vi "Load SVG Image (Path).vi"(8 "error in (no error)":errorcluster, 10 "Scale (1)":dbl=1.0, 11 "Path In":path) -> (0 "error out":errorcluster, 2 "Image":T1, 3 "Path Out":path)   [LabVIEW 2020, in "G-Image.lvlib"]
doc: "Load a Scalable Vector Graphics (SVG) image file from disk, and return it as a LabVIEW picture. The SVG is loaded assuming using 96 DPI and px units. Use the <b>Scale</b> input to adjust the size of the image being loaded.\n\nThe input can be a standard path type, a UTF-8 encoded path string, or a byte array."
uses:
  G-Image.lvlib
  <vilib>/picture/picture.llb/imagedata.ctl
  Private/Debug Path.vi
  Private/Result To Error.vi
  <vilib>/Utility/file.llb/Application Directory.vi
  <vilib>/Utility/error.llb/Error Cluster From Error Code.vi
  Private/Copy Image To Picture.vi
  Private/Get Image Data Size.vi
  <vilib>/picture/picture.llb/Create Mask By Alpha.vi
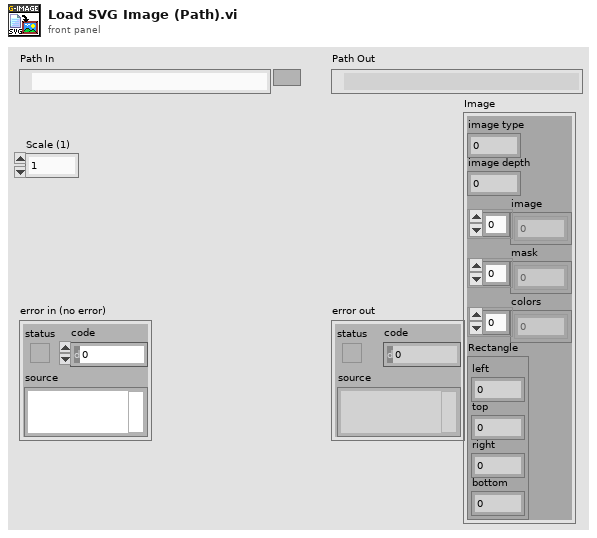
[diagram p1: front panel]
types:
  T1 = typedef "imagedata.ctl" = cluster{"image type":i32, "image depth":i32, "image":u8[], "mask":u8[], "colors":u32[], "Rectangle":cluster{"left":i16, "top":i16, "right":i16, "bottom":i16}}
  T2 = typedef "G-Image.lvlib/Extended Image.ctl" = cluster{"Image":T1, "Layers":i32, "Delays":i32[]}
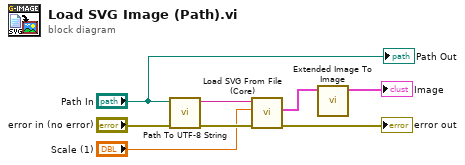
[diagram p0: block diagram]
diagram:
  n1 = call "Path To UTF-8 String.vi"("error in"="error in (no error)", "Path"="Path In") -> ("error out"=w4:errorcluster, "UTF-8 String"=w7:string)  [unwired: 8 in]
  n2 = call "Load SVG From File (Core).vi"("error in (no error)"=w4, "Scale (1)"="Scale (1)", "Path In"=w7) -> ("error out"=→"error out":errorcluster, "Extended Image"=w2:T2)  [unwired: 6 in, 1 out]
  n3 = call "Extended Image To Image.vi"("Extended Image"=w2) -> ("Image"=→"Image":T1)  [unwired: 10 in]
  "Path Out" <- "Path In"
